vi "DetectPosition(SubVI).vi"(1 "index":i32, 2 "Valley Position":dbl[](array[numeric]), 3 "Peak Position":dbl[](array[numeric]), 4 "Buffer":dbl[](array[numeric])) -> (0 "Data":dbl[](array[numeric]))   [LabVIEW 2017]
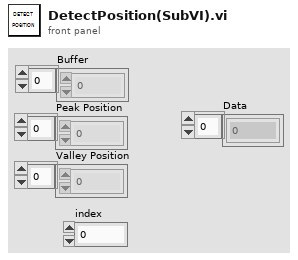
[diagram p1: front panel]
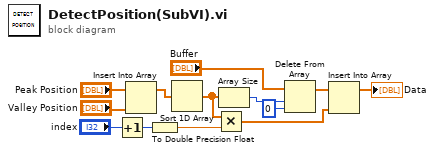
[diagram p0: block diagram]
diagram:
  n1 = Increment(x="index") -> (x+1=w4:i32)
  n2 = Insert Into Array(array="Peak Position", new element="Valley Position") -> (w6:dbl[])  [unwired: 1 in]
  n3 = To Double Precision Float(number=w4) -> (double precision float=w3:dbl)
  n4 = Sort 1D Array(array=w6) -> (sorted array=w2:dbl[])
  n5 = Multiply(x=w2, y=w3) -> (x*y=w1:dbl[])
  n6 = Array Size(array=w2) -> (size(s)=w13:i32)
  n7 = Delete From Array(array="Buffer", length=w13, index=0 ("인덱스")) -> (array with subset deleted=w11:dbl[])  [unwired: 1 out]
  n8 = Insert Into Array(array=w11, new element=w1) -> (→"Data":dbl[])  [unwired: 1 in]
